vi "runtest empty test input.vi"() -> (0 "Test Panel Input":T1={"Test Configuration (\"\")"="", "Test Execution Settings"={"Quick Mode (T)"=FALSE, "Seq Count"=0, "Step Info"="", "Instruments on Station"=[], "LANGUAGE"="English", "Files Found?"=FALSE, "Step Number"=1}, "Fields"=[]} {"Test Execution Settings"."Step Number" min=1 step=1})   [LabVIEW 2011]
uses:
  runtest test Input.ctl
  tests/Test Execution Settings.ctl
  server/database/Stations/Instruments/Instrument Record.ctl
  server/database/Fields/Field Record.ctl
  server/database/Fields/Field DataTypes.ctl
  server/database/Fields/Field NextItem.ctl
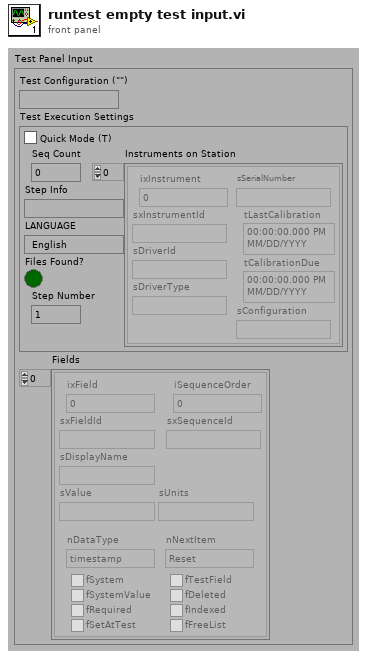
[diagram p1: front panel]
types:
  T1 = typedef "runtest test Input.ctl" = cluster{"Test Configuration (\"\")":string, "Test Execution Settings":T2, "Fields":T4[]}
  T2 = typedef "Test Execution Settings.ctl" = cluster{"Quick Mode (T)":bool, "Seq Count":i32, "Step Info":string, "Instruments on Station":T3[], "LANGUAGE":string, "Files Found?":bool, "Step Number":i32}
  T3 = typedef "Instrument Record.ctl" = cluster{"ixInstrument":i32, "sxInstrumentId":string, "sDriverId":string, "sDriverType":string, "sSerialNumber":string, "tLastCalibration":timestamp, "tCalibrationDue":timestamp, "sConfiguration":string}
  T4 = typedef "Field Record.ctl" = cluster{"ixField":i32, "iSequenceOrder":i32, "sxFieldId":string, "sxSequenceId":string, "sDisplayName":string, "sValue":string, "sUnits":string, "nDataType":T5, "nNextItem":T6, "fSystem":bool, "fSystemValue":bool, "fRequired":bool, "fSetAtTest":bool, "fTestField":bool, "fDeleted":bool, "fIndexed":bool, "fFreeList":bool}
  T5 = typedef "Field DataTypes.ctl" = enum32{"text", "numeric", "list", "timestamp", "boolean"}
  T6 = typedef "Field NextItem.ctl" = enum32{"Reset", "Retain", "Auto-Increment"}
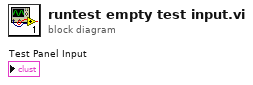
[diagram p0: block diagram]
diagram:
